vi "Synthetic_Jet_Initial.vi"() -> ()   [LabVIEW 2011]
uses:
  Controls/SJ_Data_Cluster.ctl
  Controls/SJ_Channels.ctl
  ADAM Client/Sub VIs/ADAM Controls/Update_scan_value.ctl
  Globals/Meas_global.vi
  Acquisition/Data_Translation/DataTranslation_global.vi
  <vilib>/Analysis/1siggen.llb/Ramp Pattern by Delta.vi
  <vilib>/gmath/interp.llb/Create Mesh Grid (2D) (x,y arrays).vi
  <vilib>/Analysis/NI_AALBase.lvlib
  <vilib>/gmath/NI_Gmath.lvlib
panel:
  out "Amplitude":dbl[](array[numeric])
  out "Frequency":dbl[](array[numeric])
  in  "SJ Setup Cluster":T1={"Min Amp"=1.0, "Max Amp"=1.0, "Amp Delta"=1.0, "Dwell (ms)"=100, "Min Freq"=500.0, "Max Freq"=1200.0, "Freq Delta"=10.0, "Samps/cycle"=30.0, "Optimise Target"=10.0, "No. of Iterations"=5.0, "Optimise Switch"=2, "Jet or Disc ID"=0, "Phase Average?"=TRUE, "Coefficient"=1.0} {"Optimise Switch" items=["Velocity", "Pressure", "None"]}
  in  "SJ_Data_Cluster":T2={"Do"=0.0055, "Dc"=0.038, "Ho"=0.01, "Hc"=0.008, "K"=1.14, "beta"=0.4244, "Vc"=0.0002, "Vo"=2.375829444e-07}
  out "Num of Blocks":i32=203
  in  "Device Name":refnum<visa-resource-name>="USB0::0x0699::0x0347::C036837::INSTR"
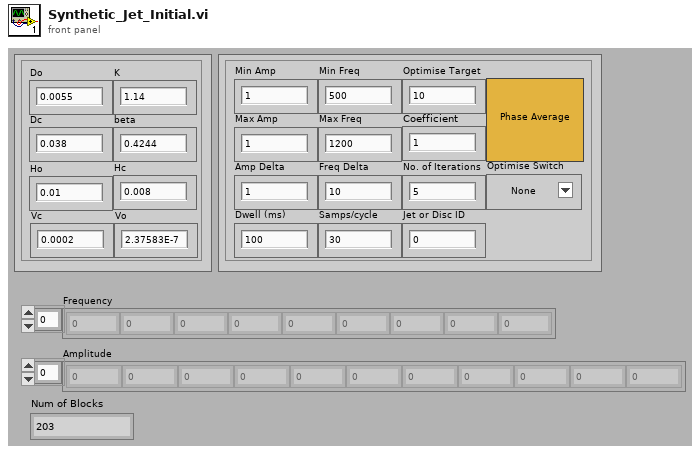
[diagram p1: front panel]
types:
  T1 = cluster{"Min Amp":dbl, "Max Amp":dbl, "Amp Delta":dbl, "Dwell (ms)":u32, "Min Freq":dbl, "Max Freq":dbl, "Freq Delta":dbl, "Samps/cycle":dbl, "Optimise Target":dbl, "No. of Iterations":dbl, "Optimise Switch":u16, "Jet or Disc ID":u32, "Phase Average?":bool, "Coefficient":dbl}
  T2 = typedef "SJ_Data_Cluster.ctl" = cluster{"Do":dbl, "Dc":dbl, "Ho":dbl, "Hc":dbl, "K":dbl, "beta":dbl, "Vc":dbl, "Vo":dbl}
  T3 = typedef "Post_Process.ctl" = enum16{"Take New Data", "Post Process Raw Data File"}
  T4 = typedef "SJ_Channels.ctl" = string[]
  T5 = typedef "Update_scan_value.ctl" = cluster{"Channel Name":string, "New Value":dbl}
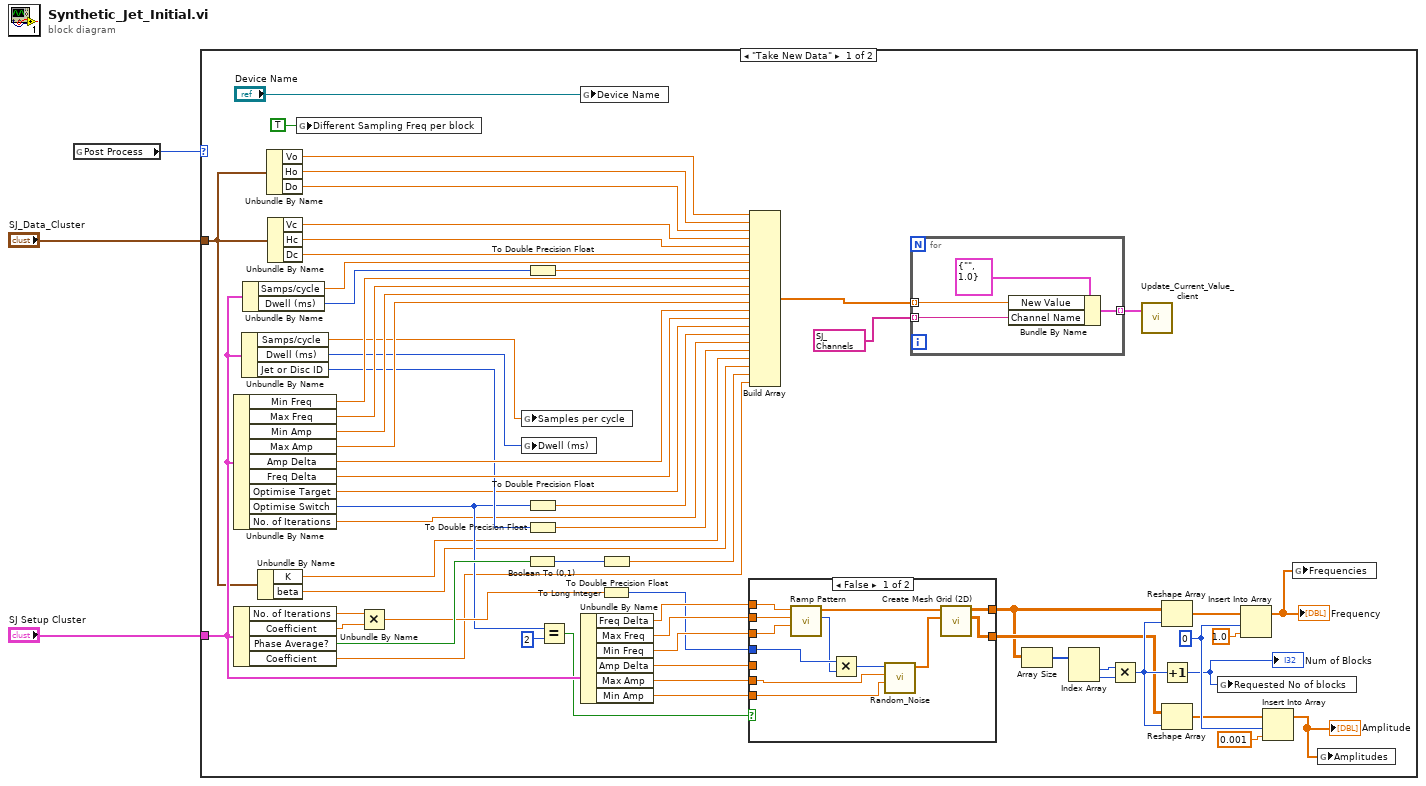
[diagram p0: block diagram]
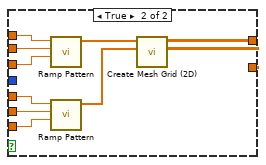
[diagram p2: hidden frame]
diagram:
  n1 = global read "Meas_global.vi" "Post Process"() -> (w1:T3)
  n2 = case shown="\"Take New Data\"" w1 {
    tunnel: "SJ Setup Cluster" -> [w41 _]
    tunnel: "SJ_Data_Cluster" -> [w31 _]
    frame "Take New Data" {
      w28 = 0 ("index")
      n3 = Unbundle By Name(w41) -> ("Min Freq"=w55:dbl, "Max Freq"=w54:dbl, "Min Amp"=w53:dbl, "Max Amp"=w52:dbl, "Amp Delta"=w51:dbl, "Freq Delta"=w50:dbl, "Optimise Target"=w34:dbl, "Optimise Switch"=w12:u16, "No. of Iterations"=w10:dbl)
      n4 = Unbundle By Name(w41) -> ("No. of Iterations"=w13:dbl, "Coefficient"=w14:dbl, "Phase Average?"=w43:bool, "Coefficient"=w9:dbl)
      n5 = Unbundle By Name(w41) -> ("Samps/cycle"=w48:dbl, "Dwell (ms)"=w49:u32, "Jet or Disc ID"=w44:u32)
      n6 = Unbundle By Name(w41) -> ("Samps/cycle"=w57:dbl, "Dwell (ms)"=w56:u32)
      n7 = Unbundle By Name(w31) -> ("K"=w6:dbl, "beta"=w7:dbl)
      n8 = Unbundle By Name(w31) -> ("Vo"=w63:dbl, "Ho"=w62:dbl, "Do"=w61:dbl)
      n9 = Unbundle By Name(w31) -> ("Vc"=w60:dbl, "Hc"=w59:dbl, "Dc"=w58:dbl)
      n10 = global write "DataTranslation_global.vi" "Different Sampling Freq per block"(TRUE ("Different Sampling Freq per block")) -> ()
      n11 = Multiply(x=w13, y=w14) -> (x*y=w30:dbl)
      n12 = global write "DataTranslation_global.vi" "Samples per cycle"(w48) -> ()
      n13 = global write "DataTranslation_global.vi" "Dwell (ms)"(w49) -> ()
      n14 = Boolean To (0,1)(Boolean=w43) -> (0, 1=w42:i16)
      n15 = To Double Precision Float(number=w56) -> (double precision float=w47:dbl)
      n16 = To Double Precision Float(number=w12) -> (double precision float=w11:dbl)
      n17 = To Double Precision Float(number=w44) -> (double precision float=w5:dbl)
      n18 = Equal?(x=w12, y=u16 2) -> (x = y?=w32:bool)
      n19 = global write "DataTranslation_global.vi" "Device Name"("Device Name") -> ()
      n20 = Unbundle By Name(w41) -> ("Freq Delta"=w40:dbl, "Max Freq"=w39:dbl, "Min Freq"=w38:dbl, "Amp Delta"=w37:dbl, "Max Amp"=w36:dbl, "Min Amp"=w35:dbl)
      n21 = To Long Integer(number=w30) -> (32bit integer=w29:i32)
      n22 = To Double Precision Float(number=w42) -> (double precision float=w8:dbl)
      n23 = case shown="False" w32 {
        tunnel: w40 -> [w77 w85]
        tunnel: w39 -> [w76 w84]
        tunnel: w38 -> [w75 w83]
        tunnel: w37 -> [_ w82]
        tunnel: w36 -> [w73 w81]
        tunnel: w35 -> [w72 w80]
        tunnel: w29 -> [w74 _]
        tunnel: [w67 w79] -> w18
        tunnel: [w66 w78] -> w19
        frame False {
          n24 = call-poly <vilib>:"Ramp Pattern.vi"("start"=w75, "end"=w76, "delta"=w77) -> ("samples"=w71:i32, "Ramp Pattern"=w69:dbl[])  [unwired: 6 in, 1 out]
          n25 = Multiply(x=w74, y=w71) -> (x*y=w70:i32)
          n26 = call "Random_Noise.vi"("min"=w72, "max"=w73, "samples"=w70) -> ("Random Noise"=w68:dbl[])  [unwired: 8 in]
          n27 = call-poly <vilib>:"Create Mesh Grid (2D).vi"("y domain"=w68, "x domain"=w69) -> ("Y"=w66:dbl[][], "X"=w67:dbl[][])  [unwired: 7 in, 1 out]
        }
        frame True {
          n28 = call-poly <vilib>:"Ramp Pattern.vi"("start"=w83, "end"=w84, "delta"=w85) -> ("Ramp Pattern"=w86:dbl[])  [unwired: 6 in, 2 out]
          n29 = call-poly <vilib>:"Ramp Pattern.vi"("start"=w80, "end"=w81, "delta"=w82) -> ("Ramp Pattern"=w87:dbl[])  [unwired: 6 in, 2 out]
          n30 = call-poly <vilib>:"Create Mesh Grid (2D).vi"("y domain"=w87, "x domain"=w86) -> ("Y"=w78:dbl[][], "X"=w79:dbl[][])  [unwired: 7 in, 1 out]
        }
      }
      n31 = Build Array(w63, w62, w61, w60, w59, w58, w57, w47, w55, w54, w53, w52, w51, w50, w34, w11, w10, w5, w6, w7, w8, w9) -> (w46:dbl[])
      n32 = for {
        tunnel: w46 -> [w90] mode=indexing
        tunnel: T4 ["Synthetic_Jet:Orifice:Volume", "Synthetic_Jet:Orifice:Height", "Synthetic_Jet:Orifice:Diameter", "Synthetic_Jet:Cavity:Volume", "Synthetic_Jet:Cavity:Height", "Synthetic_Jet:Cavity:Diameter", "Synthetic_Jet:Samples:Per_Cycle", "Synthetic_Jet:Dwell:Time", "Synthetic_Jet:Minimum:Frequency", "Synthetic_Jet:Maximum:Frequency", "Synthetic_Jet:Minimum:Amplitude", "Synthetic_Jet:Maximum:Amplitude", "Synthetic_Jet:Amplitude:Delta", "Synthetic_Jet:Frequency:Delta", "Synthetic_Jet:Calibration:Velocity", "Synthetic_Jet:Calibration:Type", "Synthetic_Jet:Calibration:No_Of_Gens", "Synthetic_Jet:Identification:Number", "Synthetic_Jet:LEM_Pressure:Coefficient", "Synthetic_Jet:LEM_Added_Mass:Coefficient", "Synthetic_Jet:Phase:Average?", "Synthetic_Jet:Optimisation:Coefficient"] ("Synthetic Jet Specific Channels") -> [w89] mode=indexing
        tunnel: [w88] -> w45 mode=indexing
        n33 = Bundle By Name(cluster=T5 {"Channel Name"="", "New Value"=1.0} ("Update Scan Value Cluster"), "New Value"=w90, "Channel Name"=w89) -> (w88:T5)
      }
      n34 = Array Size(array=w18) -> (size(s)=w20:i32[])
      n35 = Index Array(array=w20) -> (element #1=w22:i32, element #2=w21:i32)  [unwired: 2 in]
      n36 = Multiply(x=w22, y=w21) -> (x*y=w23:i32)
      n37 = call "Update_Current_Value_client.vi"("Update array in"=w45) -> ()  [unwired: 1 in]
      n38 = Reshape Array(w18, w23) -> (w24:dbl[])
      n39 = Increment(x=w23) -> (x+1=w17:i32)
      "Num of Blocks" <- w17
      n40 = Reshape Array(w19, w23) -> (w26:dbl[])
      n41 = global write "Meas_global.vi" "Requested No of blocks"(w17) -> ()
      n42 = Insert Into Array(array=w24, index=w28, new element=1.0 ("new element/subarray")) -> (w16:dbl[])
      "Frequency" <- w16
      n43 = Insert Into Array(array=w26, index=w28, new element=0.001 ("new element/subarray")) -> (w15:dbl[])
      "Amplitude" <- w15
      n44 = global write "DataTranslation_global.vi" "Frequencies"(w16) -> ()
      n45 = global write "DataTranslation_global.vi" "Amplitudes"(w15) -> ()
    }
    frame "Post Process Raw Data File" {
    }
  }
